vi "Reset Banana.vi"(8 "error in":errorcluster, 11 "Variety Configured":string) -> (0 "error out":errorcluster, 3 "Variety":string)   [LabVIEW 2021, in "Bananas.lvlib"]
uses:
  Bananas.lvlib
  Banana/Banana.lvclass
  Platano/Platano.lvclass
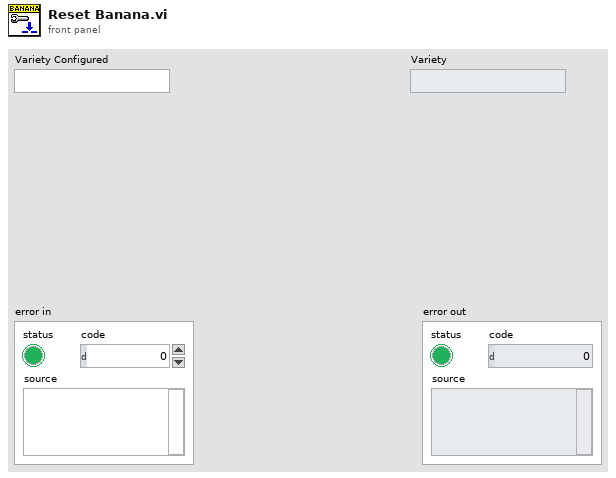
[diagram p1: front panel]
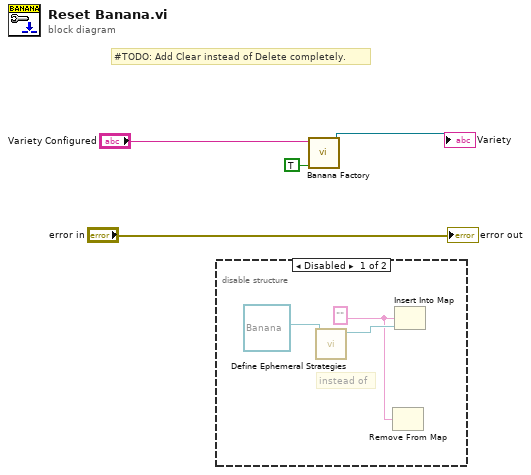
[diagram p0: block diagram]
diagram:
  # "#TODO: Add Clear instead of Delete completely."
  n1 = disable-structure shown="Disabled" {
    frame Disabled {
      w5 = ""
      # "instead of"
      n2 = call "Define Ephemeral Strategies.vi"("Platano"=refnum<class "Banana.lvclass"> refnum ("Banana")) -> ("Platano"=w6:refnum<class "Platano.lvclass">)  [unwired: 9 in, 1 out]
      n3 = Remove From Map(10:w5) -> ()  [unwired: 1 in, 3 out]
      n4 = Insert Into Map(key=w5, value=w6) -> ()  [unwired: 1 in, 3 out]
    }
    frame Enabled {
    }
  }
  n5 = call "Banana Factory.vi"("Varietal"=TRUE ("Clear"), "Platano"="Variety Configured") -> ("Banana"=→"Variety":refnum<class "Banana.lvclass">)  [unwired: 9 in]
  "error out" <- "error in"
